vi "GetS System Color.vi"(8 "错误输入（无错误）":errorcluster, 11 "SysColor":T1 items=["COLOR_SCROLLBAR"=0, "COLOR_BACKGROUND"=1, "COLOR_ACTIVECAPTION"=2, "COLOR_INACTIVECAPTION"=3, "COLOR_MENU"=4, "COLOR_WINDOW"=5, "COLOR_WINFRAME"=6, "COLOR_MENUTEXT"=7, "COLOR_WINDOWTEXT"=8, "COLOR_CAPTIONTEXT"=9, "COLOR_ACTIVEBORDER"=10, "COLOR_INACTIVEBORDER"=11, "COLOR_APPWORKSPACE"=12, "COLOR_HILIGHT"=13, "COLOR_HIGHLIGHTTEXT"=14, "COLOR_BTNFACE"=15, "COLOR_BTNSHADOW"=16, "COLOR_GRAYTEXT"=17, "COLOR_BTNTEXT"=18, "COLOR_INACTIVECAPTIONTEXT"=19, "COLOR_BTNHIGHLIGHT"=20, "COLOR_3DDKSHADOW"=21, "COLOR_3DLIGHT"=22, "COLOR_INFOTEXT"=23, "COLOR_INFORBK"=24, "COLOR_HOTLIGHT"=26, "COLOR_GRADIENTACTIVECAPTION"=27, "COLOR_GRADIENTINACTIVECAPTION"=28, "COLOR_MENUHILIGHT"=29, "COLOR_MENUBAR"=30]) -> (0 "错误输出":errorcluster, 3 "color out":u32(colorbox)=255 caption="颜色输出")   [LabVIEW 2011]
uses:
  SysteColor.ctl
  user32.dll
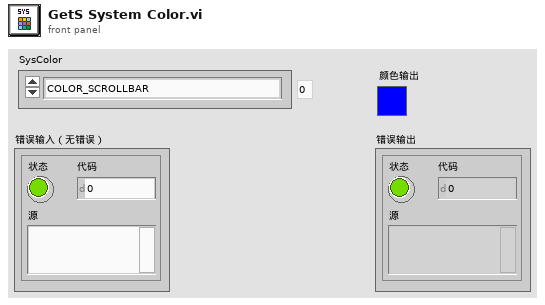
[diagram p1: front panel]
types:
  T1 = typedef "SysteColor.ctl" = i32
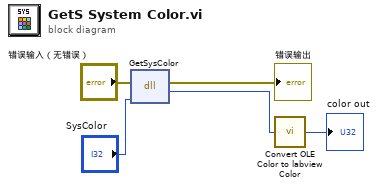
[diagram p0: block diagram]
diagram:
  n1 = dll-call lib="user32.dll" fn="GetSysColor"(error in="错误输入（无错误）", "nIndex"="SysColor") -> (error out=→"错误输出":errorcluster, "return type"=w4:u32)  [unwired: 3 in, 1 out]
  n2 = call "Convert OLE Color to labview Color.vi"("color in"=w4) -> ("color out"=→"color out":u32)
